vi "gripper information.vi"(0 "gripper":T1, 1 "Type":enum16{"Z", "I", "O", "S", "L", "J", "T", "N"}(ring)=enum."O") -> (2 "dy":dbl, 3 "dx":dbl, 4 "Angel":dbl)   [LabVIEW 2018]
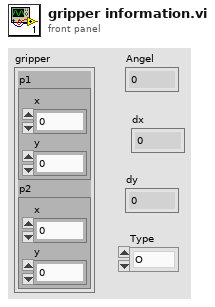
[diagram p1: front panel]
types:
  T1 = cluster{"p1":cluster{"x":dbl, "y":dbl}, "p2":cluster{"x":dbl, "y":dbl}}
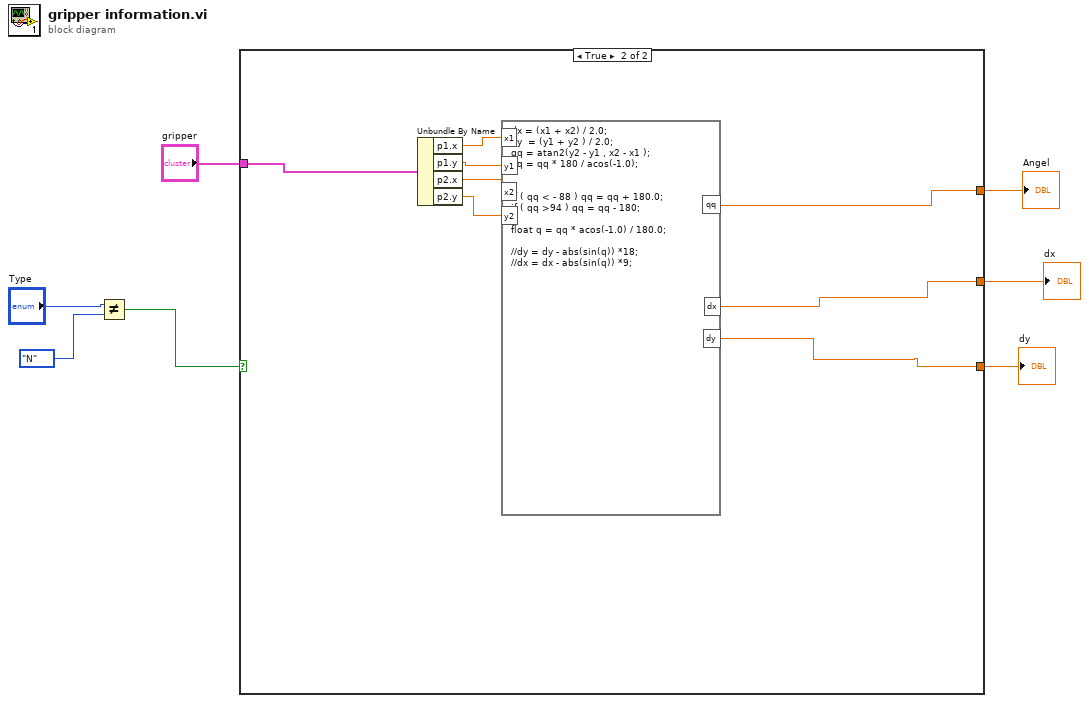
[diagram p0: block diagram]
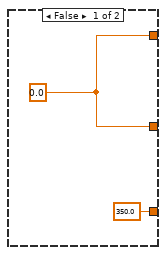
[diagram p2: hidden frame]
diagram:
  n1 = Not Equal?(x="Type", y=enum16{"Z", "I", "O", "S", "L", "J", "T", "N"}."N") -> (x != y?=w5:bool)
  n2 = case shown="True" w5 {
    tunnel: "gripper" -> [_ w13]
    tunnel: [w9 w12] -> w3
    tunnel: [w9 w11] -> w2
    tunnel: [350.0 ("dy") w10] -> w1
    frame False {
      w9 = 0.0
    }
    frame True {
      n3 = Unbundle By Name(w13) -> ("p1.x"=w17:dbl, "p1.y"=w16:dbl, "p2.x"=w15:dbl, "p2.y"=w14:dbl)
      n4 = formula code="dx = (x1 + x2) / 2.0;\ndy  = (y1 + y2 ) / 2.0;\nqq = atan2(y2 - y1 , x2 - x1 );\nqq = qq * 180 / acos(-1.0);\n\n\nif ( qq < - 88 ) qq = qq + 180.0;\nif ( qq >94 ) qq = qq - 180;\n\nfloat q = qq * acos(-1.0) / 180.0;\n\n//dy = dy - abs(sin(q)) *18;\n//dx = dx - abs(sin(q)) *9;"("x1"=w17, "y1"=w16, "x2"=w15, "y2"=w14) -> ("qq"=w12:dbl, "dx"=w11:dbl, "dy"=w10:dbl)
    }
  }
  "Angel" <- w3
  "dx" <- w2
  "dy" <- w1
